vi "Get Class Names.vi"(8 "error in (no error)":errorcluster, 11 "Scan Driver in":refnum<class "Scan Driver.lvclass">) -> (0 "error out":errorcluster, 1 "Reader name":string, 2 "Scanner name":string, 3 "Scan Driver out":refnum<class "Scan Driver.lvclass">)   [LabVIEW 2009, in "Scan Driver.lvclass"]
doc: "Get the .lvclass names of the Scanner and Reader inside this Scan Driver instance (perhaps for writing to a file.)"
uses:
  Scan Driver.lvclass
  Scan Driver.lvclass/Scan Driver.ctl
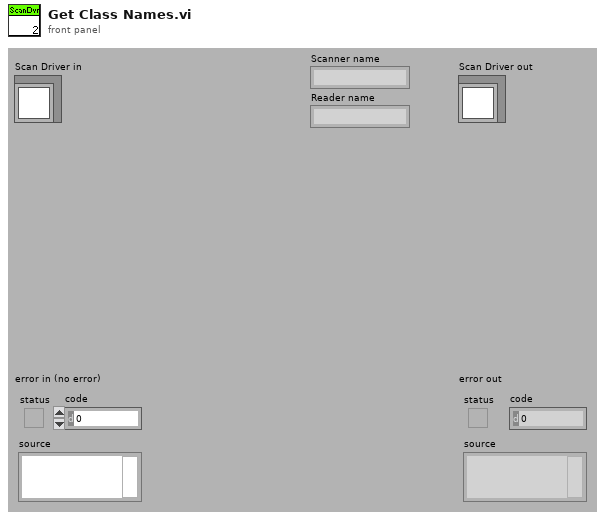
[diagram p1: front panel]
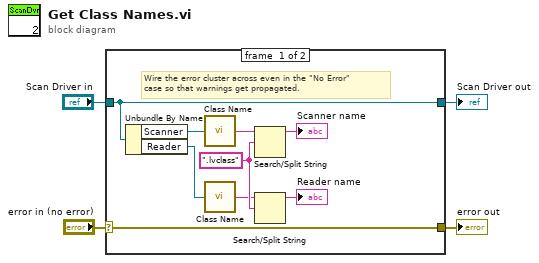
[diagram p0: block diagram]
diagram:
  n1 = case shown="No Error" "error in (no error)" {
    selector: "error in (no error)" -> [w13 w15]
    tunnel: [w13 w15] -> w3
    tunnel: [w12 w14] -> w1
    tunnel: "Scan Driver in" -> [w12 w14]
    frame #0 {
      w9 = ".lvclass" ("search string/char (-)")
      # "Wire the error cluster across even in the \"No Error\"\ncase so that warnings get propagated."
      n2 = Unbundle By Name(w12) -> ("Scanner"=w11:refnum<class "Scanner.lvclass">, "Reader"=w10:refnum<class "Reader.lvclass">)
      n3 = call "Class Name.vi"("LabVIEW Object"=w11) -> ("Classname"=w7:string)
      n4 = call "Class Name.vi"("LabVIEW Object"=w10) -> ("Classname"=w8:string)
      n5 = Search/Split String(string=w7, search string/char (-)=w9) -> (substring before match=→"Scanner name":string)  [unwired: 3 out]
      n6 = Search/Split String(string=w8, search string/char (-)=w9) -> (substring before match=→"Reader name":string)  [unwired: 3 out]
    }
    frame #1 {
    }
  }
  "error out" <- w3
  "Scan Driver out" <- w1
